vi "Set Loop Rate with Refs.vi"(6 "Target Rate":dbl=1000.0, 8 "error in (no error)":errorcluster, 10 "Targets":refnum<k24>[](array[refnum]), 11 "Sysdef":refnum<k24>) -> (0 "error out":errorcluster)   [LabVIEW 2011]
uses:
  NationalInstruments.VeriStand.SystemDefinitionAPI
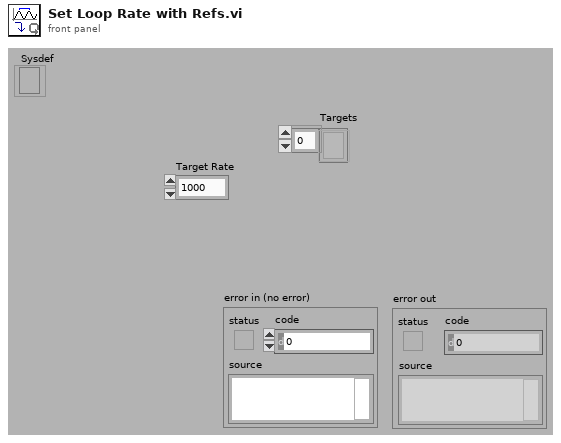
[diagram p1: front panel]
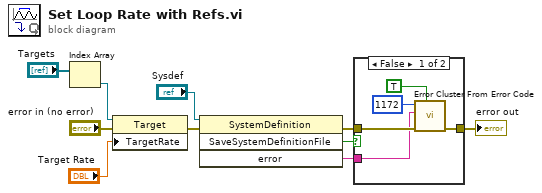
[diagram p0: block diagram]
diagram:
  n1 = Index Array(array="Targets") -> (element=w7:refnum<k24>)  [unwired: 1 in]
  n2 = property class="Target"(reference=w7, error in="error in (no error)", "TargetRate"="Target Rate") -> (error out=w6:errorcluster)  [unwired: 1 out]
  n3 = invoke class="SystemDefinition" method="SaveSystemDefinitionFile"(reference="Sysdef", error in=w6) -> (error out=w2:errorcluster, "SaveSystemDefinitionFile"=w4:bool, "error"=w1:string)  [unwired: 2 in, 1 out]
  n4 = case shown="False" w4 {
    tunnel: [w14 w16] -> w3
    tunnel: w2 -> [w15 w16]
    tunnel: w1 -> [w12 _]
    frame False {
      n5 = call <vilib>:"Error Cluster From Error Code.vi"("show call chain? (False)"=TRUE, "error in (no error)"=w15, "error message (\"\")"=w12, "error code (0)"=1172) -> ("error out"=w14:errorcluster)  [unwired: 5 in]
    }
    frame True {
    }
  }
  "error out" <- w3
